vi "networkStreamLoop.vi"(5 "JSON cmd queue":refnum<queue>, 7 "Control Data Notifier":refnum<notifier>, 8 "error in":errorcluster, 9 "Message Queues":T2, 10 "Processed Data Notifier":refnum<notifier>, 11 "daqRefDes":string) -> (0 "error out":errorcluster)   [LabVIEW 2024]
uses:
  Message Queue/All Message Queues.ctl
  Message Queue/Message Cluster.ctl
  Control/StreamCluster_TypeDef.ctl
  Control/Array Data Constant.ctl
  Control/Control Data Constant.ctl
  Control/streamIO_states.ctl
  3813366e-2ad4-4fa9-bcbf-b7f5b322ef8f.vi
  <vilib>/MediaMongrels Ltd/WebSockets/Sockets/VISA TCP Socket/VISA TCP.lvclass
  C:/Program Files/National Instruments/LabVIEW 2024/vi.lib/MediaMongrels Ltd/WebSockets/Sockets/Socket/Socket.lvclass
  Globals.vi
  <vilib>/JDP Science/JSONtext/Variant to JSON Text.vi
  <vilib>/ErrorRing/Error Ring.xnode
  <vilib>/JDP Science/JSONtext/LVClass Serializer/JSONtext LVClass Serializer.lvclass
  <vilib>/MediaMongrels Ltd/WebSockets/WebSockets/WebSocket Server/WebSocket Server.lvclass
  Message Queue/Message Queue.lvlib
  <vilib>/JDP Science/JSONtext/JSONtext.lvlib
panel:
  out "Network Steam Iteration Clock (ms)":u32
  out "Network Stream Loop Iteration Counter":i32
  in  "StreamCluster_TypeDef":T1={"DAQ"={"ManagmentRate_Hz"=1000, "StreamRate_Hz"=10, "StreamRate_ms"=0, "ManagmentRate_ms"=1000, "refDesArray"=[]}, "Modules"=[]}
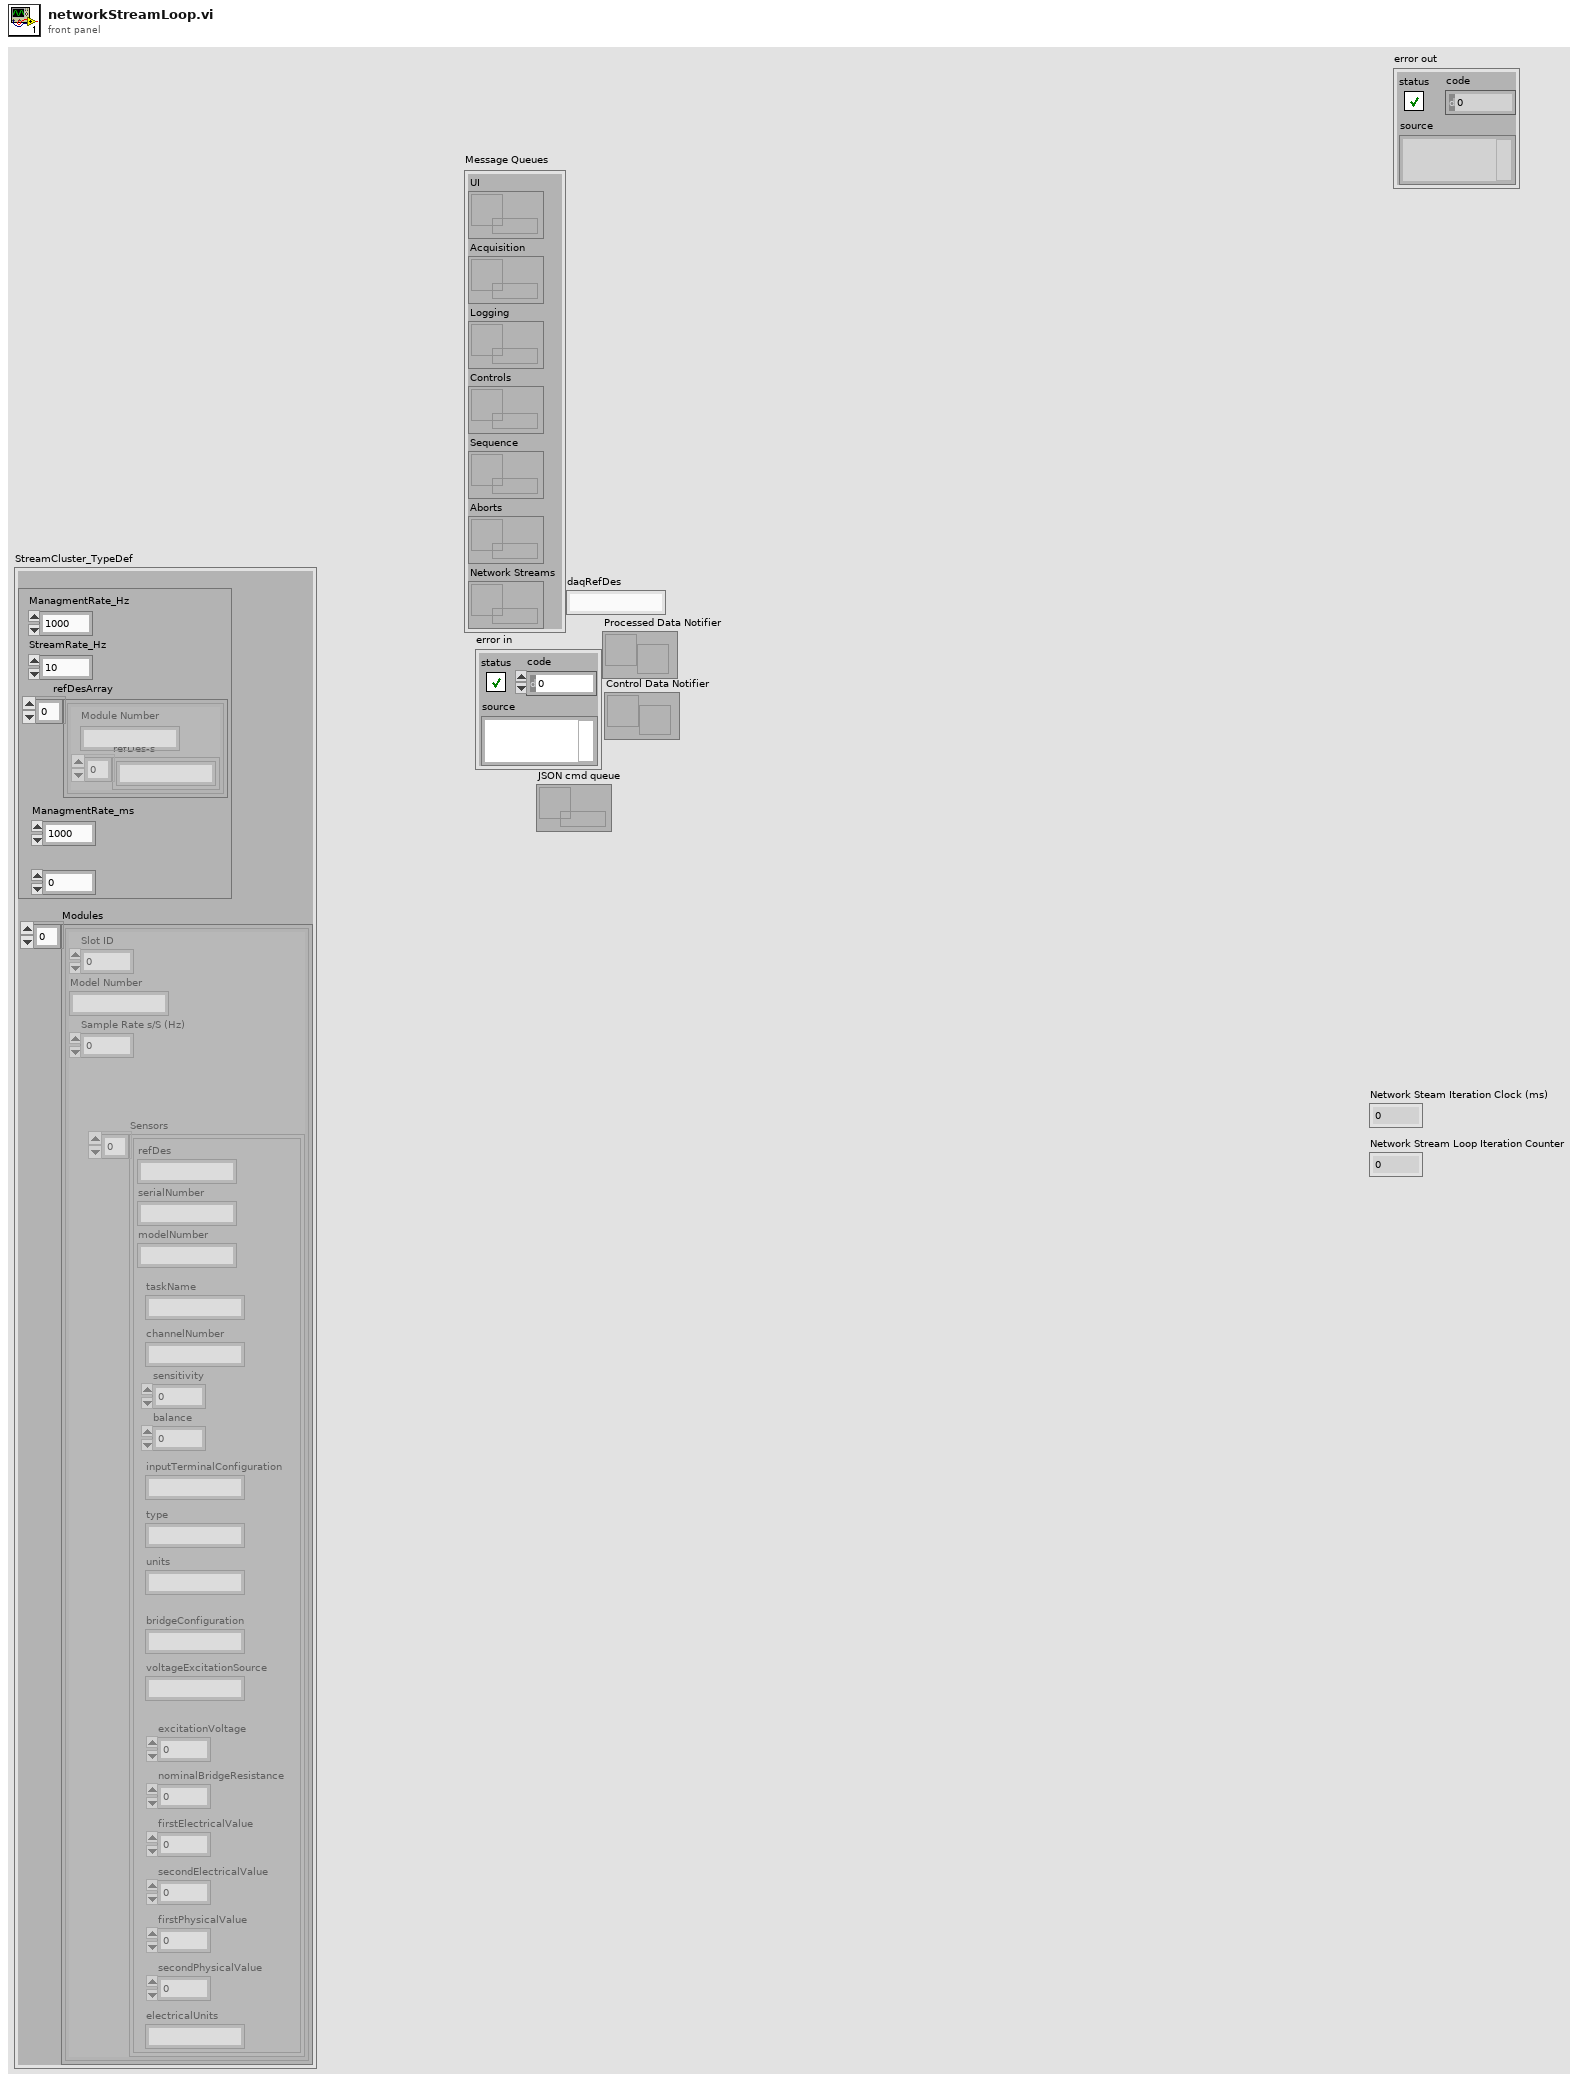
[diagram p1: front panel]
types:
  T1 = typedef "StreamCluster_TypeDef.ctl" = cluster{"DAQ":cluster{"ManagmentRate_Hz":i32, "StreamRate_Hz":i32, "StreamRate_ms":i32, "ManagmentRate_ms":i32, "refDesArray":cluster{"refDes-s":string[], "Module Number":string}[]}, "Modules":cluster{"Slot ID":i32, "Model Number":string, "Sample Rate s/S (Hz)":dbl, "Sensors":cluster{"refDes":string, "serialNumber":string, "modelNumber":string, "units":string, "balance":dbl, "sensitivity":dbl, "type":string, "inputTerminalConfiguration":string, "channelNumber":string, "taskName":string, "bridgeConfiguration":string, "excitationVoltage":dbl, "voltageExcitationSource":string, "nominalBridgeResistance":dbl, "firstElectricalValue":dbl, "secondElectricalValue":dbl, "firstPhysicalValue":dbl, "secondPhysicalValue":dbl, "electricalUnits":string}[]}[]}
  T2 = typedef "Message Queue.lvlib/All Message Queues.ctl" = cluster{"UI":refnum<queue>, "Acquisition":refnum<queue>, "Logging":refnum<queue>, "Controls":refnum<queue>, "Sequence":refnum<queue>, "Aborts":refnum<queue>, "Network Streams":refnum<queue>}
  T3 = typedef "streamIO_states.ctl" = enum16{"Fault", "Initialize", "Stream", "Close"}
  T4 = typedef "Array Data Constant.ctl" = cluster{"AI":dbl[], "TC":dbl[], "BC":dbl[], "DI":dbl[], "t (UTC)":dbl}
  T5 = typedef "Control Data Constant.ctl" = cluster{"Time (utc)":ext, "Data Out":cluster{"DO":bool[], "Module Number":string}[]}
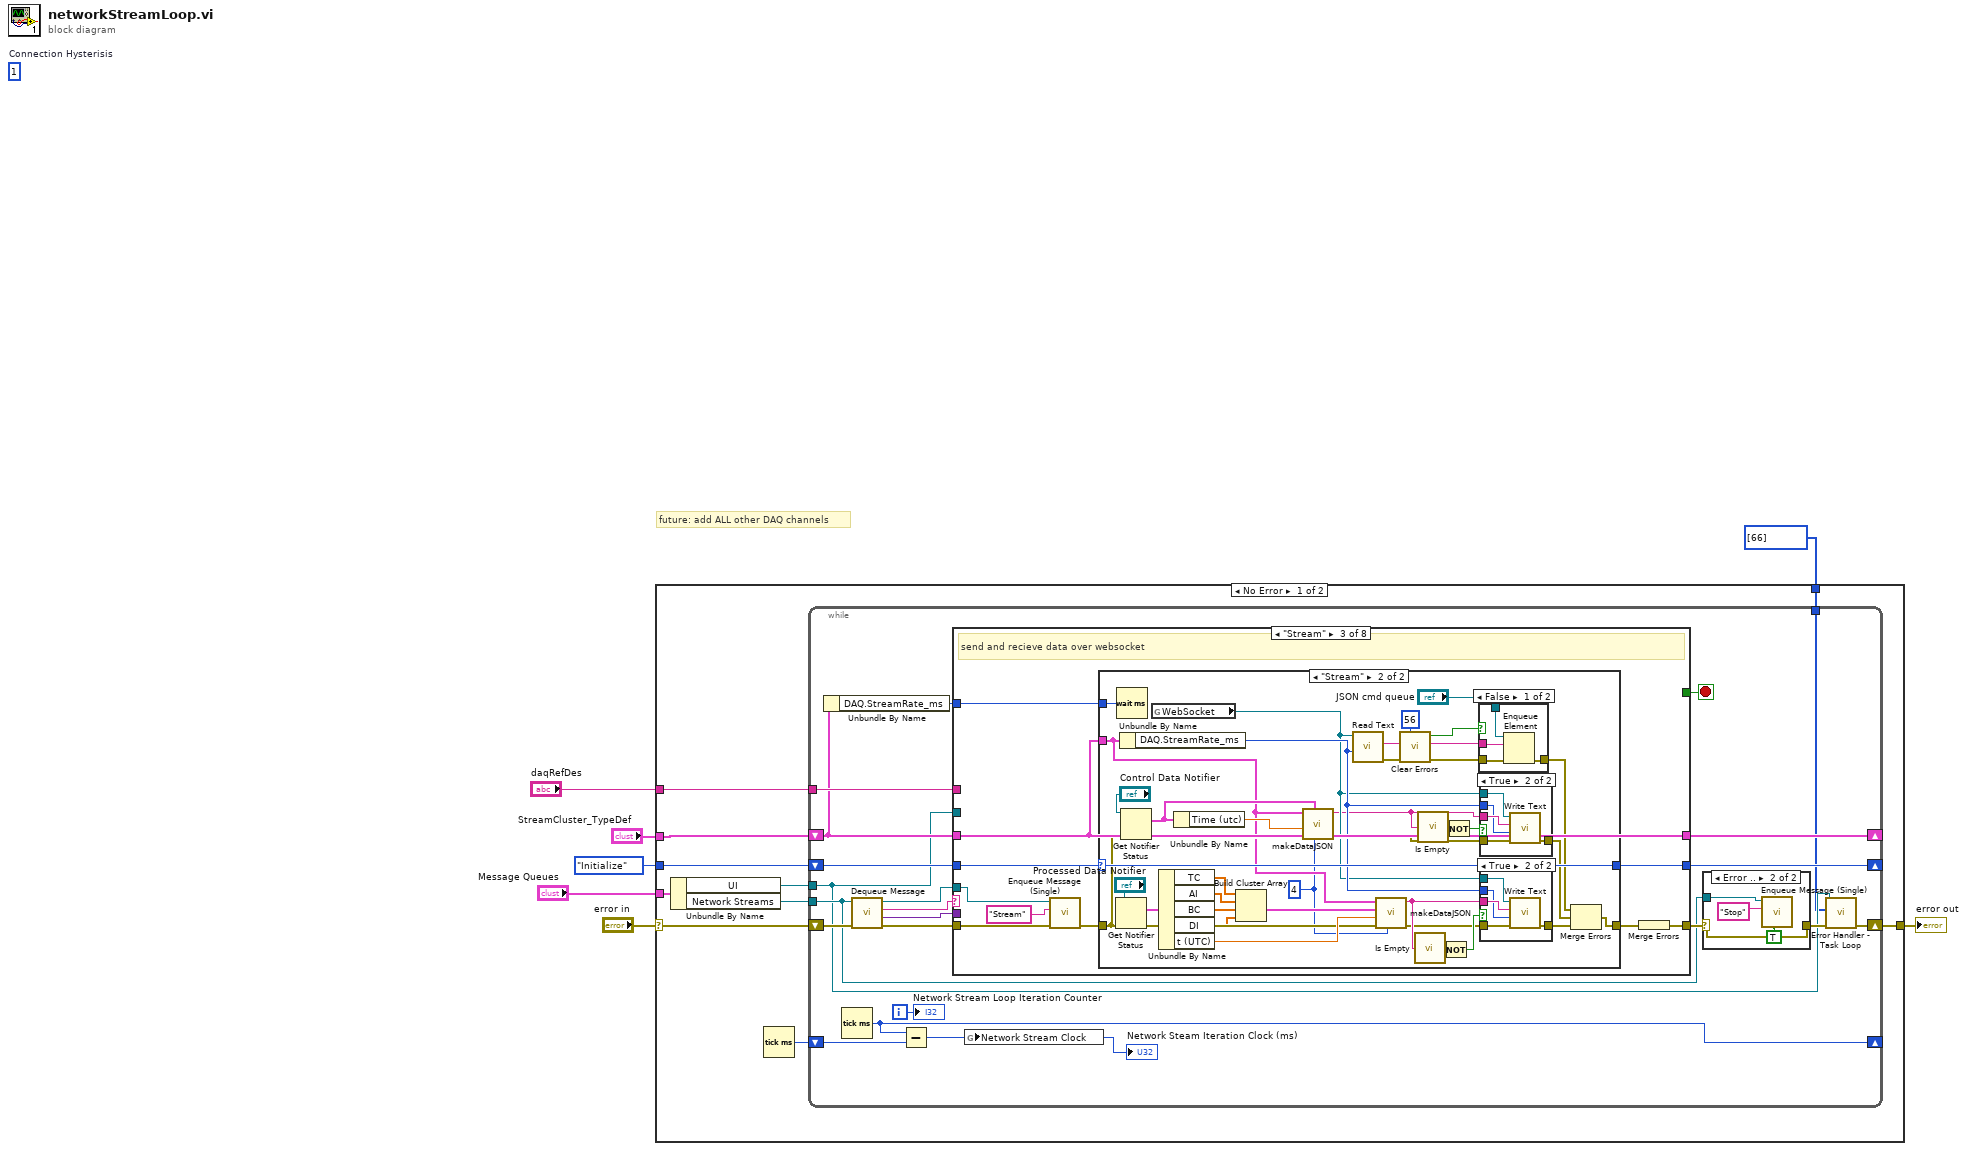
[diagram p0: block diagram]
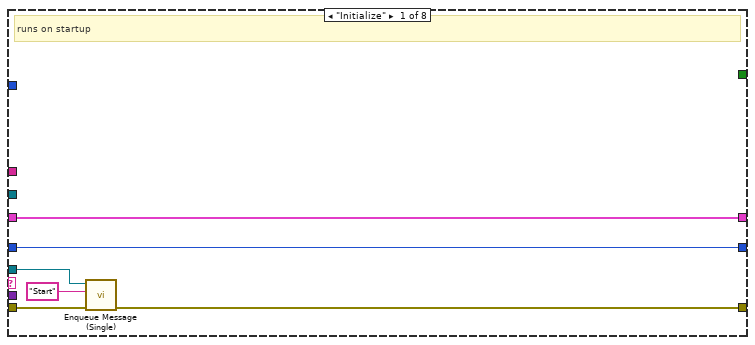
[diagram p3: hidden frame]
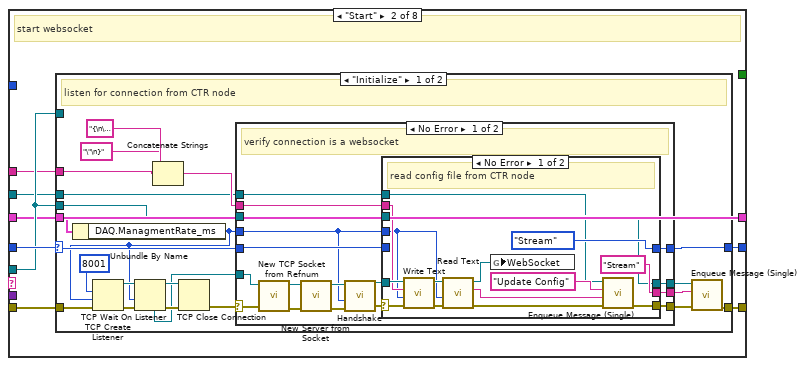
[diagram p4: hidden frame]
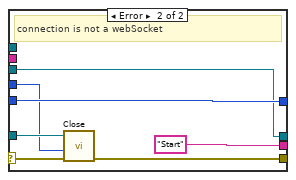
[diagram p5: hidden frame]
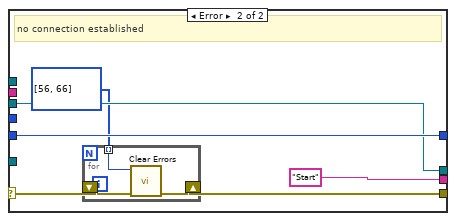
[diagram p6: hidden frame]
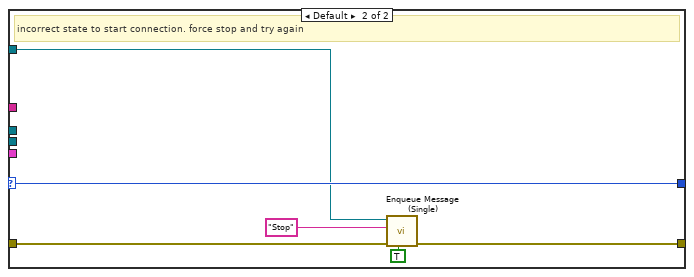
[diagram p7: hidden frame]
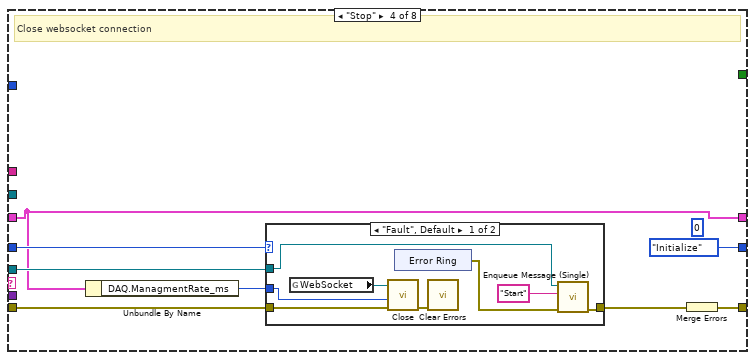
[diagram p12: hidden frame]
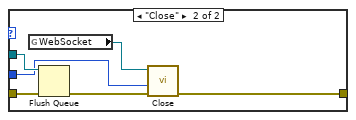
[diagram p13: hidden frame]
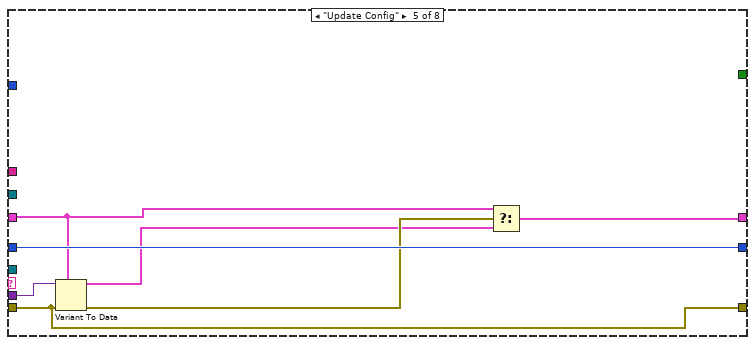
[diagram p14: hidden frame]
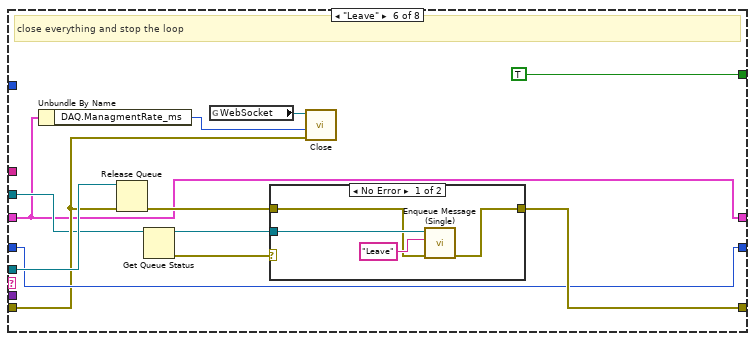
[diagram p15: hidden frame]
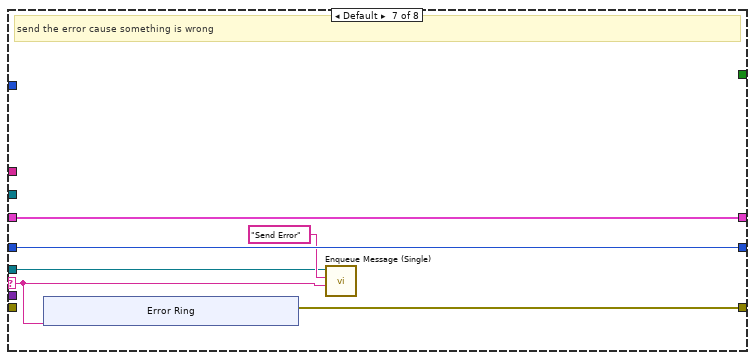
[diagram p17: hidden frame]
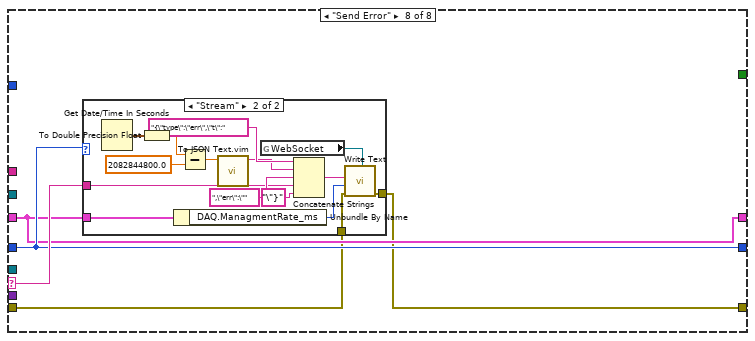
[diagram p18: hidden frame]
diagram:
  (unwired) 1  # Connection Hysterisis
  # "future: add ALL other DAQ channels"
  n1 = case shown="No Error" "error in" {
    selector: "error in" -> [w17 w281]
    tunnel: "Message Queues" -> [w15 _]
    tunnel: [w16 w281] -> w4
    tunnel: "StreamCluster_TypeDef" -> [w9 _]
    tunnel: streamIO_states."Initialize" ("stream state") -> [w11 _]
    tunnel: "daqRefDes" -> [w10 _]
    tunnel: i32[] [66] ("Ignore Errors (Runtime)") -> [w8 _]
    frame No Error {
      n2 = Unbundle By Name(w15) -> ("UI"=w13:refnum<queue>, "Network Streams"=w14:refnum<queue>)
      n3 = Tick Count (ms)() -> (millisecond timer value=w12:u32)
      n4 = while {
        shift-right: [w34] -> w16
        shift-left: w17 -> [w39]
        tunnel: w14 -> [w22]
        tunnel: w13 -> [w20]
        shift-right: [w33] -> _
        shift-left: w11 -> [w27]
        shift-right: [w30] -> _
        shift-left: w12 -> [w31]
        shift-right: [w24] -> _
        shift-left: w9 -> [w21]
        tunnel: w10 -> [w23]
        tunnel: w8 -> [w19]
        i -> [w29]
        stop <- w32 stop-if-true
        n5 = Unbundle By Name(w21) -> ("DAQ.StreamRate_ms"=w18:i32)
        n6 = Tick Count (ms)() -> (millisecond timer value=w30:u32)
        n7 = call "Dequeue Message.vi"("error in (no error)"=w39, "Message Queue"=w22) -> ("error out"=w35:errorcluster, "Message Data"=w36:variant, "Message"=w37:string, "dup Message Queue"=w38:refnum<queue>)  [unwired: 6 in]
        n8 = Subtract(x=w30, y=w31) -> (x-y=w28:u32)
        "Network Steam Iteration Clock (ms)" <- w28
        n9 = case shown="\"Stream\"" w37 {
          selector: w37 -> [_ _ _ _ _ _ w251 w264]
          tunnel: w38 -> [w48 w54 w137 w209 _ w243 w249 _]
          tunnel: w36 -> [_ _ _ _ w231 _ _ _]
          tunnel: w35 -> [w45 w57 w138 w208 w229 w236 _ w260]
          tunnel: w20 -> [_ w51 _ _ _ w234 _ _]
          tunnel: [w49 w56 w144 w207 w229 w242 w252 w261] -> w26
          tunnel: [w50 w58 w141 streamIO_states."Initialize" ("stream state") w230 w237 w254 w263] -> w33
          tunnel: [_ _ _ _ _ TRUE _ _] -> w32
          tunnel: w27 -> [w50 w55 w142 w206 w230 w237 w254 w263]
          tunnel: w21 -> [w46 w52 w140 w203 w225 w233 w253 w262]
          tunnel: [w46 w52 w140 w203 w228 w233 w253 w262] -> w24
          tunnel: w23 -> [_ w53 _ _ _ _ _ _]
          tunnel: w18 -> [_ _ w135 _ _ _ _ _]
          frame "Initialize" {
            # "runs on startup"
            n10 = call "Enqueue Message (Single).vi"("error in (no error)"=w45, "Message"="Start", "Message Queue"=w48) -> ("error out"=w49:errorcluster)  [unwired: 7 in, 1 out]
          }
          frame "Start" {
            # "start websocket"
            n11 = case shown="\"Initialize\"" w55 {
              selector: w55 -> [w70 w134]
              tunnel: [w71 w134] -> w58
              tunnel: w57 -> [w77 w132]
              tunnel: w54 -> [_ w130]
              tunnel: [w80 w131] -> w56
              tunnel: w54 -> [w68 _]
              tunnel: w53 -> [w63 _]
              tunnel: w52 -> [w62 _]
              tunnel: w51 -> [w60 _]
              frame "Initialize" {
                # "listen for connection from CTR node"
                n12 = Unbundle By Name(w62) -> ("DAQ.ManagmentRate_ms"=w61:i32)
                n13 = TCP Create Listener(8:w77, 9:w61, 10:u16 8001 ("port")) -> (0:w79:errorcluster, 3:w76:refnum<k5>)  [unwired: 2 in, 1 out]
                n14 = TCP Wait On Listener(8:w79, 9:w61, 11:w76) -> (0:w78:errorcluster, 3:w75:refnum<k5>, 4:w73:refnum<k5>)  [unwired: 1 in, 2 out]
                n15 = Concatenate Strings("{\n\"type\": \"config_req\", \n\"refDes\": \"", w63, "\"\n}") -> (w64:string)
                n16 = TCP Close Connection(connection ID=w75, error in (no error)=w78) -> (error out=w74:errorcluster)  [unwired: 1 in, 1 out]
                n17 = case shown="No Error" w74 {
                  selector: w74 -> [w93 w122]
                  tunnel: w73 -> [w92 _]
                  tunnel: [w89 w121] -> w72
                  tunnel: [w88 w125] -> w71
                  tunnel: w70 -> [w87 w125]
                  tunnel: [w86 "Start"] -> w69
                  tunnel: w68 -> [w85 w123]
                  tunnel: w64 -> [w84 _]
                  tunnel: [w83 w123] -> w67
                  tunnel: w61 -> [w82 _]
                  tunnel: w60 -> [w81 _]
                  frame No Error {
                    # "verify connection is a websocket"
                    n18 = call <vilib>:"New TCP Socket from Refnum.vi"("error in (no error)"=w93, "TCP Network Connection Refnum"=w92) -> ("error out"=w95:errorcluster, "VISA TCP out"=w94:refnum<class "VISA TCP.lvclass">)  [unwired: 8 in]
                    n19 = call <vilib>:"New Server from Socket.vi"("error in (no error)"=w95, "Socket"=w94) -> ("error out"=w96:errorcluster, "WebSocket Server out"=w97:refnum<class "WebSocket Server.lvclass">)  [unwired: 8 in]
                    n20 = call-dynamic "Handshake.vi"("error in (no error)"=w96, "timeout ms (5000)"=w82, "WebSocket Connection in"=w97) -> ("error out"=w91:errorcluster, "WebSocket Connection out"=w90:refnum<class "WebSocket Server.lvclass">)  [unwired: 7 in]
                    n21 = case shown="No Error" w91 {
                      selector: w91 -> [w102 w119]
                      tunnel: w90 -> [w103 w118]
                      tunnel: [w109 w117] -> w89
                      tunnel: [streamIO_states."Stream" ("stream state") w116] -> w88
                      tunnel: w87 -> [_ w116]
                      tunnel: ["Stream" "Start"] -> w86
                      tunnel: w85 -> [w99 w114]
                      tunnel: w84 -> [w101 _]
                      tunnel: [w99 w114] -> w83
                      tunnel: w82 -> [w100 w113]
                      tunnel: w81 -> [w98 _]
                      frame No Error {
                        # "read config file from CTR node"
                        n22 = call-dynamic "Write Text.vi"("error in (no error)"=w102, "timeout ms (5000)"=w100, "String Data"=w101, "WebSocket in"=w103) -> ("error out"=w105:errorcluster, "WebSocket out"=w104:refnum<class "WebSocket Server.lvclass">)  [unwired: 6 in]
                        n23 = call-dynamic "Read Text.vi"("error in (no error)"=w105, "timeout ms (5000)"=w100, "WebSocket in"=w104) -> ("error out"=w108:errorcluster, "Data"=w107:string, "WebSocket out"=w110:refnum<class "WebSocket Server.lvclass">)  [unwired: 6 in]
                        n24 = global write "Globals.vi" "WebSocket"(w110) -> ()
                        n25 = call "Enqueue Message (Single).vi"("error in (no error)"=w108, "Message Data"=w107, "Message"="Update Config", "Message Queue"=w98) -> ("error out"=w109:errorcluster)  [unwired: 6 in, 1 out]
                      }
                      frame Error {
                        # "connection is not a webSocket"
                        n26 = call-dynamic "Close.vi"("error in (no error)"=w119, "timeout ms (5000)"=w113, "WebSocket in"=w118) -> ("error out"=w117:errorcluster)  [unwired: 8 in]
                      }
                    }
                  }
                  frame Error {
                    # "no connection established"
                    n27 = for {
                      shift-right: [w127] -> w121
                      shift-left: w122 -> [w128]
                      tunnel: i32[] [56, 66] -> [w126] mode=indexing
                      n28 = call <vilib>:"Clear Errors.vi"("error in (no error)"=w128, "specific error code to clear (0: all)"=w126) -> ("error out"=w127:errorcluster)  [unwired: 4 in, 1 out]
                    }
                  }
                }
                n29 = call "Enqueue Message (Single).vi"("error in (no error)"=w72, "Message"=w69, "Message Queue"=w67) -> ("error out"=w80:errorcluster)  [unwired: 7 in, 1 out]
              }
              frame Default {
                # "incorrect state to start connection. force stop and try again"
                n30 = call "Enqueue Message (Single).vi"("Priority Message? (F)"=TRUE, "error in (no error)"=w132, "Message"="Stop", "Message Queue"=w130) -> ("error out"=w131:errorcluster)  [unwired: 6 in, 1 out]
              }
            }
          }
          frame "Stream" {
            # "send and recieve data over websocket"
            n31 = call "Enqueue Message (Single).vi"("error in (no error)"=w138, "Message"="Stream", "Message Queue"=w137) -> ("error out"=w136:errorcluster)  [unwired: 7 in, 1 out]
            n32 = case shown="\"Stream\"" w142 {
              selector: w142 -> [w145 w184]
              tunnel: w136 -> [w146 w169]
              tunnel: [w146 w181] -> w143
              tunnel: [w145 w184] -> w141
              tunnel: w140 -> [_ w150]
              tunnel: w135 -> [_ w151]
              frame Default {
              }
              frame "Stream" {
                w148 = 4
                n33 = Get Notifier Status(notifier="Processed Data Notifier", error in (no error)=w169) -> (current notification=w178:T4, error out=w168:errorcluster)  [unwired: 3 out]
                n34 = Wait (ms)(milliseconds to wait=w151) -> ()  [unwired: 1 out]
                n35 = Unbundle By Name(w150) -> ("DAQ.StreamRate_ms"=w163:i32)
                n36 = Get Notifier Status(notifier="Control Data Notifier", error in (no error)=w169) -> (current notification=w166:T5, error out=w167:errorcluster)  [unwired: 3 out]
                n37 = global read "Globals.vi" "WebSocket"() -> (w162:refnum<class "WebSocket Server.lvclass">)
                n38 = Unbundle By Name(w178) -> ("TC"=w175:dbl[], "AI"=w174:dbl[], "BC"=w177:dbl[], "DI"=w156:dbl[], "t (UTC)"=w176:dbl)
                n39 = Unbundle By Name(w166) -> ("Time (utc)"=w165:ext)
                n40 = Build Cluster Array(w175, w174, w177, w156) -> (w149:cluster{"DI":dbl[]}[])
                n41 = call "makeDataJSON.vi"("data array size"=w148, "latest notification"=w166, "error in"=w167, "time stamp (UTC)"=w165, "StreamCluster_TypeDef"=w150) -> ("error out"=w164:errorcluster, "JSON Package"=w159:string)  [unwired: 5 in]
                n42 = call-dynamic "Read Text.vi"("timeout ms (5000)"=w163, "WebSocket in"=w162) -> ("error out"=w183:errorcluster, "Data"=w152:string)  [unwired: 7 in, 1 out]
                n43 = call "makeDataJSON.vi"("data array size"=w148, "error in"=w168, "time stamp (UTC)"=w176, "data cluster array"=w149, "StreamCluster_TypeDef"=w150) -> ("error out"=w157:errorcluster, "JSON Package"=w173:string)  [unwired: 5 in]
                n44 = call <vilib>:"Clear Errors.vi"("error in (no error)"=w183, "specific error code to clear (0: all)"=56) -> ("error out"=w155:errorcluster, "specific error cleared?"=w154:bool)  [unwired: 4 in]
                n45 = call <vilib>:"Is Empty.vi"("JSON"=w173) -> ("Empty"=w172:bool)  [unwired: 4 in]
                n46 = call <vilib>:"Is Empty.vi"("JSON"=w159) -> ("Empty"=w160:bool)  [unwired: 4 in]
                n47 = Not(x=w172) -> (.not. x?=w171:bool)
                n48 = Not(x=w160) -> (.not. x?=w161:bool)
                n49 = case shown="False" w154 {
                  tunnel: w155 -> [w186 w189]
                  tunnel: [w188 w189] -> w153
                  tunnel: w152 -> [w187 _]
                  tunnel: "JSON cmd queue" -> [w185 _]
                  frame False {
                    n50 = Enqueue Element(queue=w185, element=w187, error in (no error)=w186) -> (error out=w188:errorcluster)  [unwired: 1 in, 2 out]
                  }
                  frame True {
                  }
                }
                n51 = case shown="True" w161 {
                  tunnel: [w190 w195] -> w158
                  tunnel: w163 -> [_ w193]
                  tunnel: w162 -> [_ w192]
                  tunnel: w159 -> [_ w194]
                  tunnel: w164 -> [w190 w191]
                  frame False {
                  }
                  frame True {
                    n52 = call-dynamic "Write Text.vi"("error in (no error)"=w191, "timeout ms (5000)"=w193, "String Data"=w194, "WebSocket in"=w192) -> ("error out"=w195:errorcluster)  [unwired: 6 in, 1 out]
                  }
                }
                n53 = case shown="True" w171 {
                  tunnel: [w196 w201] -> w180
                  tunnel: w163 -> [_ w199]
                  tunnel: w162 -> [_ w198]
                  tunnel: w173 -> [_ w200]
                  tunnel: w157 -> [w196 w197]
                  frame False {
                  }
                  frame True {
                    n54 = call-dynamic "Write Text.vi"("error in (no error)"=w197, "timeout ms (5000)"=w199, "String Data"=w200, "WebSocket in"=w198) -> ("error out"=w201:errorcluster)  [unwired: 6 in, 1 out]
                  }
                }
                n55 = Merge Errors(w153, w158, w180) -> (w181:errorcluster)
              }
            }
            n56 = Merge Errors(w143) -> (w144:errorcluster)
          }
          frame "Stop" {
            (unwired) 0 ("ConnectionHysterisis")
            # "Close websocket connection"
            n57 = Unbundle By Name(w203) -> ("DAQ.ManagmentRate_ms"=w202:i32)
            n58 = case shown="\"Fault\", Default" w206 {
              tunnel: w209 -> [w213 w224]
              tunnel: w208 -> [w216 w223]
              tunnel: [w214 w221] -> w204
              tunnel: w202 -> [w210 w219]
              frame "Fault", Default {
                n59 = global read "Globals.vi" "WebSocket"() -> (w217:refnum<class "WebSocket Server.lvclass">)
                n60 = call-dynamic "Close.vi"("error in (no error)"=w216, "timeout ms (5000)"=w210, "WebSocket in"=w217) -> ("error out"=w215:errorcluster)  [unwired: 8 in]
                n61 = xnode "Error Ring"() -> ("error out"=w212:errorcluster)
                n62 = call <vilib>:"Clear Errors.vi"("error in (no error)"=w215) -> ()  [unwired: 5 in, 2 out]
                n63 = call "Enqueue Message (Single).vi"("error in (no error)"=w212, "Message"="Start", "Message Queue"=w213) -> ("error out"=w214:errorcluster)  [unwired: 7 in, 1 out]
              }
              frame "Close" {
                n64 = global read "Globals.vi" "WebSocket"() -> (w220:refnum<class "WebSocket Server.lvclass">)
                n65 = Flush Queue(queue=w224, error in (no error)=w223) -> (error out=w222:errorcluster)  [unwired: 2 out]
                n66 = call-dynamic "Close.vi"("error in (no error)"=w222, "timeout ms (5000)"=w219, "WebSocket in"=w220) -> ("error out"=w221:errorcluster)  [unwired: 8 in]
              }
            }
            n67 = Merge Errors(w204) -> (w207:errorcluster)
          }
          frame "Update Config" {
            n68 = Variant To Data(error in=w229, type=w225, Variant=w231) -> (data=w226:T1, error out=w227:errorcluster)
            n69 = Select(t=w225, s=w227, f=w226) -> (s? t:f=w228:T1)
          }
          frame "Leave" {
            # "close everything and stop the loop"
            n70 = Unbundle By Name(w233) -> ("DAQ.ManagmentRate_ms"=w232:i32)
            n71 = Release Queue(queue=w243, error in (no error)=w236) -> (error out=w239:errorcluster)  [unwired: 1 in, 2 out]
            n72 = Get Queue Status(queue=w234) -> (queue out=w240:refnum<queue>, error out=w238:errorcluster)  [unwired: 2 in, 6 out]
            n73 = global read "Globals.vi" "WebSocket"() -> (w235:refnum<class "WebSocket Server.lvclass">)
            n74 = case shown="No Error" w238 {
              tunnel: [w247 w248] -> w242
              tunnel: w240 -> [w245 _]
              tunnel: w239 -> [w244 w248]
              frame No Error {
                n75 = call "Enqueue Message (Single).vi"("error in (no error)"=w244, "Message"="Leave", "Message Queue"=w245) -> ("error out"=w247:errorcluster)  [unwired: 7 in, 1 out]
              }
              frame Error {
              }
            }
            n76 = call-dynamic "Close.vi"("error in (no error)"=w236, "timeout ms (5000)"=w232, "WebSocket in"=w235) -> ()  [unwired: 8 in, 1 out]
          }
          frame Default {
            # "send the error cause something is wrong"
            n77 = xnode "Error Ring"("parameter 0"=w251) -> ("error out"=w252:errorcluster)
            n78 = call "Enqueue Message (Single).vi"("Message Data"=w251, "Message"="Send Error", "Message Queue"=w249) -> ()  [unwired: 7 in, 2 out]
          }
          frame "Send Error" {
            n79 = case shown="\"Stream\"" w263 {
              tunnel: w264 -> [_ w275]
              tunnel: w262 -> [_ w268]
              tunnel: [w265 w267] -> w261
              tunnel: w260 -> [w265 w266]
              frame Default {
              }
              frame "Stream" {
                n80 = Get Date/Time In Seconds() -> (seconds since 1Jan1904=w272:timestamp)
                n81 = To Double Precision Float(number=w272) -> (double precision float=w271:dbl)
                n82 = Unbundle By Name(w268) -> ("DAQ.ManagmentRate_ms"=w279:i32)
                n83 = Subtract(x=w271, y=2082844800.0) -> (x-y=w273:dbl)
                n84 = call "To JSON Text.vim"("Anything"=w273) -> ("<JSON>"=w269:string)  [unwired: 9 in, 1 out]
                n85 = global read "Globals.vi" "WebSocket"() -> (w280:refnum<class "WebSocket Server.lvclass">)
                n86 = Concatenate Strings("{\"type\":\"err\",\"t\":" ("string"), w269, ",\"err\":\"" ("string"), w275, "\"}" ("string")) -> (w274:string)
                n87 = call-dynamic "Write Text.vi"("error in (no error)"=w266, "timeout ms (5000)"=w279, "String Data"=w274, "WebSocket in"=w280) -> ("error out"=w267:errorcluster)  [unwired: 6 in, 1 out]
              }
            }
          }
        }
        n88 = global write "Globals.vi" "Network Stream Clock"(w28) -> ()
        n89 = case shown="Error .." w26 {
          selector: w26 -> [w40 w41]
          tunnel: [w40 w41] -> w25
          tunnel: w22 -> [_ w44]
          frame No Error {
          }
          frame Error {
            n90 = call "Enqueue Message (Single).vi"("Priority Message? (F)"=TRUE, "Message"="Stop", "Message Queue"=w44) -> ()  [unwired: 7 in, 2 out]
          }
        }
        n91 = call "Error Handler - Task Loop.vi"("error in (no error)"=w25, "Ignore Errors (Runtime)"=w19, "Message Queue"=w20) -> ("dup error in"=w34:errorcluster)  [unwired: 7 in, 1 out]
        "Network Stream Loop Iteration Counter" <- w29
      }
    }
    frame Error {
    }
  }
  "error out" <- w4
